vi "dfd_FXP Range.vi"(9 "signed?":bool=TRUE, 10 "iwl":i16, 11 "wl":i16) -> (1 "full range":ext format="%.2f", 2 "low":ext format="%.2f", 3 "high":ext format="%.2f")   [LabVIEW 2017, in "NI_DigFilter_FXP.lvlib"]
uses:
  <vilib>/addons/Digital Filter Design/NI_DigFilter_FXP.lvlib
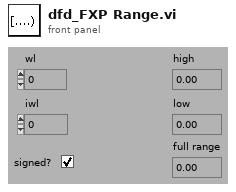
[diagram p1: front panel]
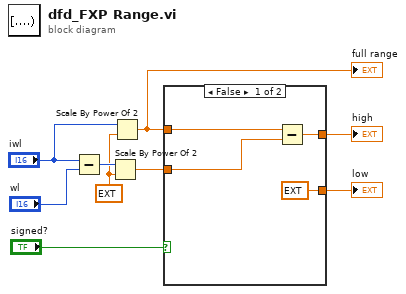
[diagram p0: block diagram]
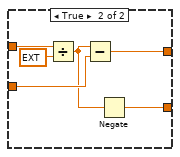
[diagram p2: hidden frame]
diagram:
  w7 = ext 1.0 ("x")
  n1 = Subtract(x="iwl", y="wl") -> (x-y=w8:i16)
  n2 = Scale By Power Of 2(n=w8, x=w7) -> (x*2^n=w4:ext)
  n3 = Scale By Power Of 2(n="iwl", x=w7) -> (x*2^n=w1:ext)
  "full range" <- w1
  n4 = case shown="False" "signed?" {
    tunnel: w1 -> [w11 w19]
    tunnel: w4 -> [w10 w17]
    tunnel: [w12 w16] -> w3
    tunnel: [ext 0.0 w14] -> w2
    frame False {
      n5 = Subtract(x=w11, y=w10) -> (x-y=w12:ext)
    }
    frame True {
      n6 = Divide(x=w19, y=ext 2.0) -> (x/y=w15:ext)
      n7 = Subtract(x=w15, y=w17) -> (x-y=w16:ext)
      n8 = Negate(x=w15) -> (-x=w14:ext)
    }
  }
  "high" <- w3
  "low" <- w2
